vi "LX-Initial Camera1.vi"(8 "error in (no error)":errorcluster caption="错误输入（无错误）") -> (0 "error out":errorcluster caption="错误输出", 2 "cam0":T1)   [LabVIEW 2017]
uses:
  <vilib>/vision/driver/NI_Vision_Acquisition_Software.lvlib
  <vilib>/vision/driver/IMAQdx.llb/IMAQdx Acquisition Mode.ctl
  <vilib>/userdefined/High Color/IMAQdx.ctl
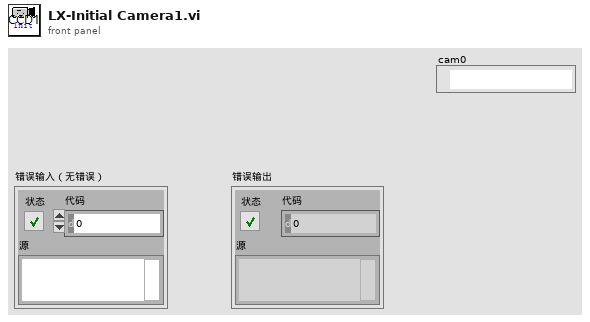
[diagram p1: front panel]
types:
  T1 = typedef "IMAQdx.ctl" = refnum<k21>
  T2 = typedef "NI_Vision_Acquisition_Software.lvlib/IMAQdx Acquisition Mode.ctl" = enum32{"One Shot", "Continuous"}
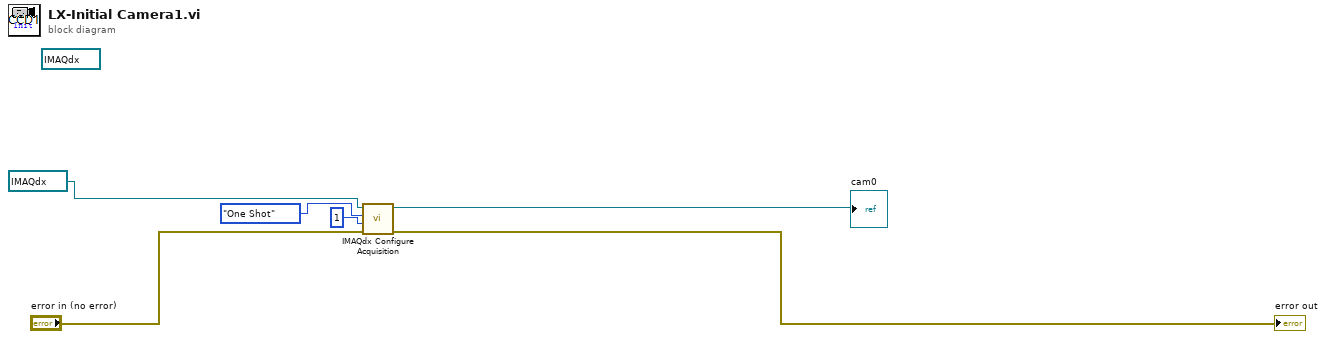
[diagram p0: block diagram]
diagram:
  (unwired) T1 "cam0" ("Session Iin")
  n1 = call <vilib>:"IMAQdx Configure Acquisition.vi"("error in"="error in (no error)", "Number of Buffers"=u32 1, "Continuous?"=IMAQdx_Acquisition_Mode."One Shot", "Session In"=T1 "cam0" ("Session Iin")) -> ("error out"=→"error out":errorcluster, "Session Out"=→"cam0":T1)  [unwired: 6 in]
